vi "Run Test.vi"(8 "error in (no error)":errorcluster, 11 "Test Template in":refnum<class "Test Template.lvclass">) -> (0 "error out":errorcluster, 1 "Positions":i32[](array[numeric]), 2 "Tests Passed":bool[](array[boolean]), 3 "Test Template out":refnum<class "Test Template.lvclass">, 5 "Fail Codes":string[](array[string]))   [LabVIEW 2015, in "Test Template.lvclass"]
uses:
  Test Template.lvclass
  Classes/Application/Class/Application.lvclass
  Test Class/Test Class.lvclass
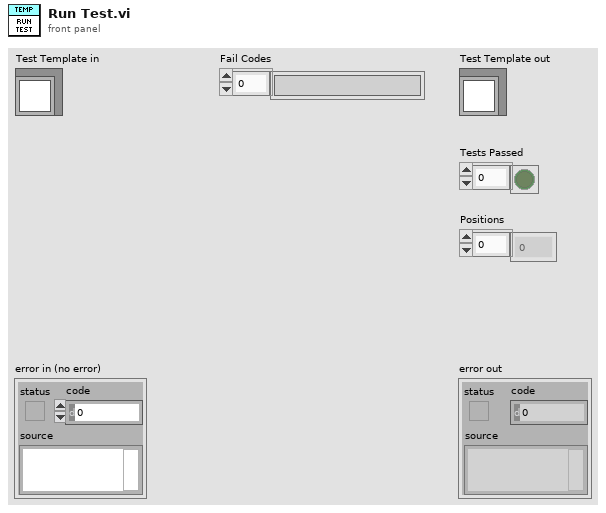
[diagram p1: front panel]
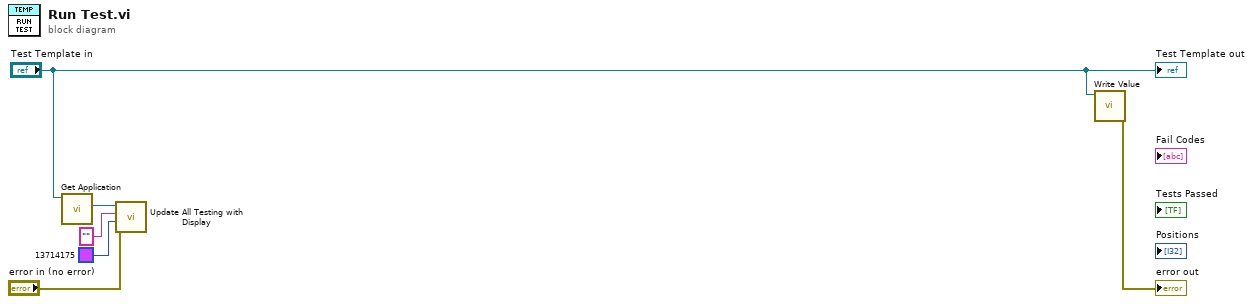
[diagram p0: block diagram]
diagram:
  n1 = call "Get Application.vi"("Test Class in"="Test Template in") -> ("Application.lvlib:Application.lvclass"=w6:refnum<class "Application.lvclass">)  [unwired: 9 in, 1 out]
  n2 = call "Update All Testing with Display.vi"("error in (no error)"="error in (no error)", "BG Color"=u32 13714175, "Message ('')"="", "Application in"=w6) -> ()  [unwired: 6 in, 2 out]
  n3 = call "Write Value.vi"("Test Class in"="Test Template in") -> ("error out"=→"error out":errorcluster)  [unwired: 10 in]
  "Test Template out" <- "Test Template in"
